vi "Write Stored Sessions.vi"(10 "Stored Sessions":refnum<class "Session.lvclass">[](array[class]), 11 "TCPConnectionHandler in":refnum<class "TCPConnectionHandler.lvclass">) -> (3 "TCPConnectionHandler out":refnum<class "TCPConnectionHandler.lvclass">)   [LabVIEW 2013, in "MQTT_TCP.lvlib" / "TCPConnectionHandler.lvclass"]
uses:
  TCPConnectionHandler.lvclass
  MQTT_Base/Session/Session.lvclass
  TCPConnectionHandler.lvclass/TCPConnectionHandler.ctl
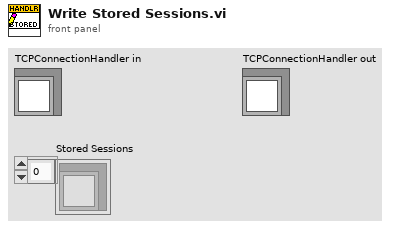
[diagram p1: front panel]
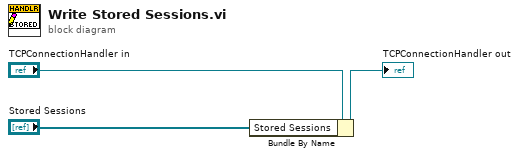
[diagram p0: block diagram]
diagram:
  n1 = Bundle By Name(cluster="TCPConnectionHandler in", "Stored Sessions"="Stored Sessions") -> (→"TCPConnectionHandler out":refnum<class "TCPConnectionHandler.lvclass">)
